vi "檔案_Timer.vi"() -> ()   [LabVIEW 2015]
panel:
  out "存檔":bool
  out "Tab Control":T1(tab)
  in  "Time Out":dbl caption="全速百分比"
  in  "機構部件":T1(ring)
  in  "Save Button":bool
  out "Recipe":string
  in  "Exit":bool
  # "Recipe - 動作延遲時間表(秒)"
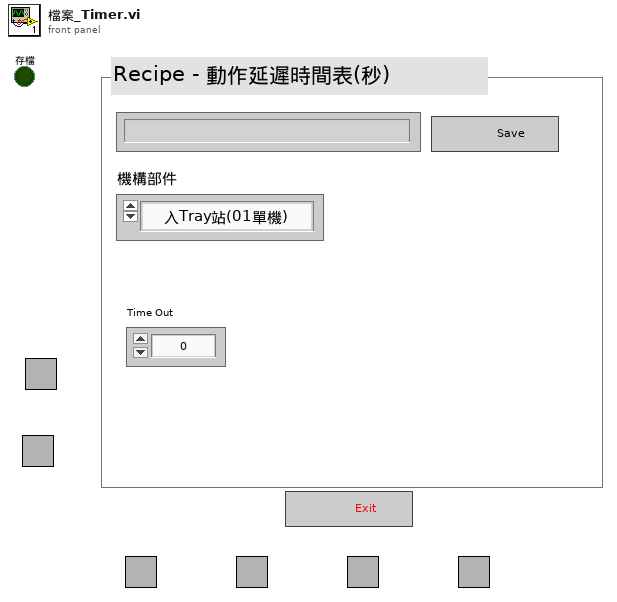
[diagram p1: front panel]
types:
  T1 = enum32{"入Tray站(01單機)", "入料站(02單機)", "對位站(02單機)", "撕膜站(03單機)", "Ag站(04單機)", "UV站(05單機)", "Folding站(06單機)", "固化站(07單機)", "噴碼站(08單機)", "出料站(09單機)", "出Tray站(10單機)", "Index站"}
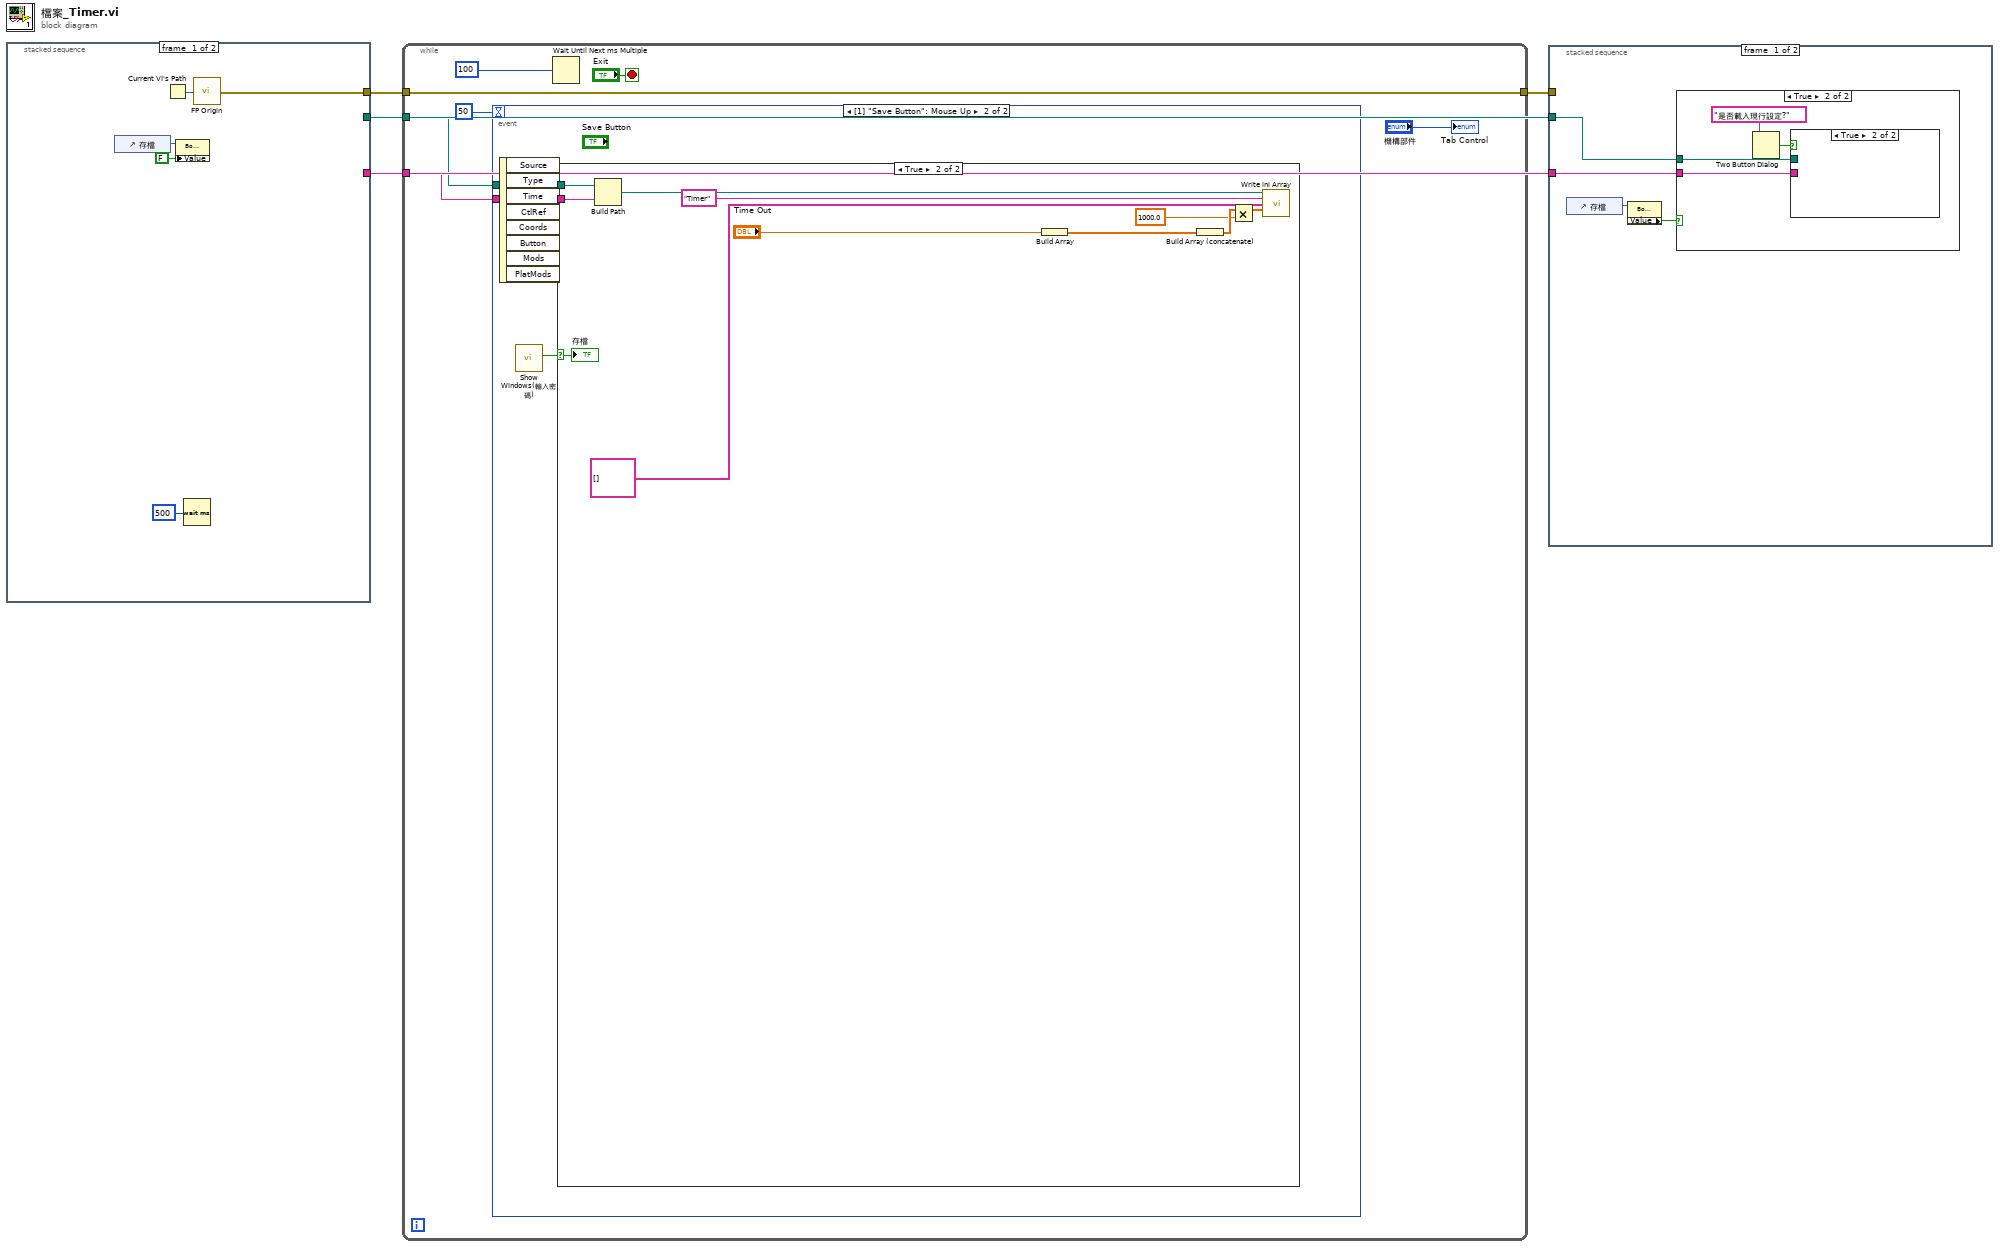
[diagram p0: block diagram]
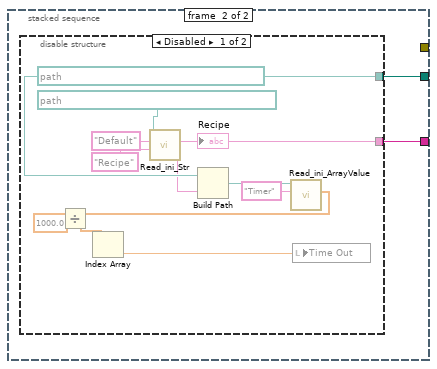
[diagram p2: hidden frame]
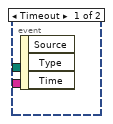
[diagram p4: hidden frame]
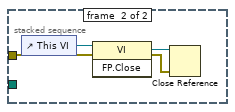
[diagram p8: hidden frame]
diagram:
  n1 = stacked-sequence {
    tunnel: [w8 _] -> w3
    tunnel: [_ w10] -> w1
    tunnel: [_ w11] -> w2
    frame #0 {
      n2 = control-ref of="存檔"() -> (w7:refnum<vi>)
      n3 = Current VI's Path() -> (path=w9:path)
      n4 = property class="Bool (strict)"(reference=w7, "Value"=FALSE) -> ()  [unwired: 1 in, 2 out]
      n5 = Wait (ms)(milliseconds to wait=u32 500) -> ()  [unwired: 1 out]
      n6 = call "FP Origin.vi"("vi path"=w9) -> ("error out"=w8:errorcluster)
    }
    frame #1 {
      n7 = disable-structure shown="Disabled" {
        disable-tunnel: [w19 _] -> w11
        disable-tunnel: [w18 _] -> w10
        frame Disabled {
          w19 = path "D:/半自動電檢機 Data/Recipe/Position" ("configuration file path")
          n8 = call "Read_ini_Str.vi"("key"="Recipe", "section"="Default", "configuration file path"=path "D:/半自動電檢機 Data/Recipe/Default.ini") -> ("value"=w18:string)  [unwired: 7 in, 1 out]
          "Recipe" <- w18
          n9 = Build Path(base path=w19, name or relative path=w18) -> (appended path=w17:path)
          n10 = call "Read_ini_ArrayValue.vi"("section"="Timer", "configuration file path"=w17) -> ("ArrayValue"=w14:dbl[])  [unwired: 8 in, 1 out]
          n11 = Divide(x=w14, y=1000.0 ("Index站_安全位確認")) -> (x/y=w13:dbl[])
          n12 = Index Array(array=w13) -> (element=w15:dbl)  [unwired: 1 in]
          n13 = local write "Time Out"(w15) -> ()
        }
        frame Enabled {
        }
      }
    }
  }
  n14 = while {
    tunnel: w3 -> [w26]
    tunnel: [w26] -> w4
    tunnel: w1 -> [w25]
    tunnel: w2 -> [w24]
    stop <- "Exit" stop-if-true
    n15 = event shown="[1] \"Save Button\": Mouse Up" {
      selector: _ -> [_ _]
      dyn-events: _ -> [_ _]
      timeout: 50 -> [_ _]
      tunnel: w25 -> [_ w32]
      tunnel: w24 -> [_ w31]
      event Timeout {
        n16 = event-data() -> ()  [unwired: 1 in, 3 out]
      }
      event "Save Button": Mouse Up {
        n17 = event-data() -> ()  [unwired: 1 in, 8 out]
        n18 = call "Show Windows(輸入密碼).vi"() -> ("密碼正確"=w30:bool)  [unwired: 10 in, 1 out]
        n19 = case shown="True" w30 {
          selector: w30 -> [_ w36]
          tunnel: w32 -> [_ w43]
          tunnel: w31 -> [_ w42]
          frame False {
          }
          frame True {
            n20 = Build Path(base path=w42, name or relative path=w43) -> (appended path=w41:path)
            n21 = Build Array("Time Out") -> (w38:dbl[])
            n22 = Build Array (concatenate)(w38) -> (w37:dbl[])
            n23 = Multiply(x=w37, y=1000.0 ("Index站_安全位確認")) -> (x*y=w35:dbl[])
            n24 = call "Write ini Array.vi"("configuration file path"=w41, "section"="Timer" ("key"), "KeysArray"=string[] [], "ValueArray"=w35) -> ()  [unwired: 11 in, 1 out]
            "存檔" <- w36
          }
        }
      }
    }
    n25 = Wait Until Next ms Multiple(millisecond multiple=u32 100) -> ()  [unwired: 1 out]
    "Tab Control" <- "機構部件"
  }
  n26 = stacked-sequence {
    tunnel: w4 -> [_ w55]
    tunnel: w2 -> [w47 _]
    tunnel: w1 -> [w46 _]
    frame #0 {
      n27 = control-ref of="存檔"() -> (w45:refnum<vi>)
      n28 = property class="Bool (strict)"(reference=w45) -> ("Value"=w44:bool)  [unwired: 1 in, 2 out]
      n29 = case shown="True" w44 {
        tunnel: w47 -> [_ w49]
        tunnel: w46 -> [_ w48]
        frame False {
        }
        frame True {
          n30 = Two Button Dialog(message="是否載入現行設定?") -> (T button?=w51:bool)  [unwired: 2 in]
          n31 = case shown="True" w51 {
            tunnel: w49 -> [_ _]
            tunnel: w48 -> [_ _]
            frame False {
            }
            frame True {
            }
          }
        }
      }
    }
    frame #1 {
      n32 = control-ref of="This VI"() -> (w54:refnum<vi>)
      n33 = invoke class="VI" method="FP.Close"(reference=w54, error in=w55) -> (reference out=w53:refnum<vi>, error out=w52:errorcluster)  [unwired: 1 in, 1 out]
      n34 = Close Reference(reference=w53, error in (no error)=w52) -> ()  [unwired: 1 out]
    }
  }
